vi "Set Tree Item Icon.vi"(0 "TreeControl in":refnum<vi>, 11 "error in (no error)":errorcluster) -> (4 "TreeControl out":refnum<vi>, 6 "Measurement folder Tags":string[](array[string]), 8 "Measurement file Tags":string[](array[string]), 15 "error out":errorcluster)   [LabVIEW 2021, in "Converter.lvlib"]
uses:
  Converter.lvlib
  0ae78c54-1542-49f1-a264-372c03cee13b.vi
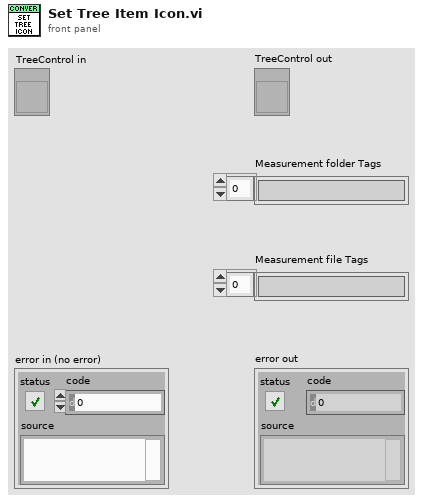
[diagram p1: front panel]
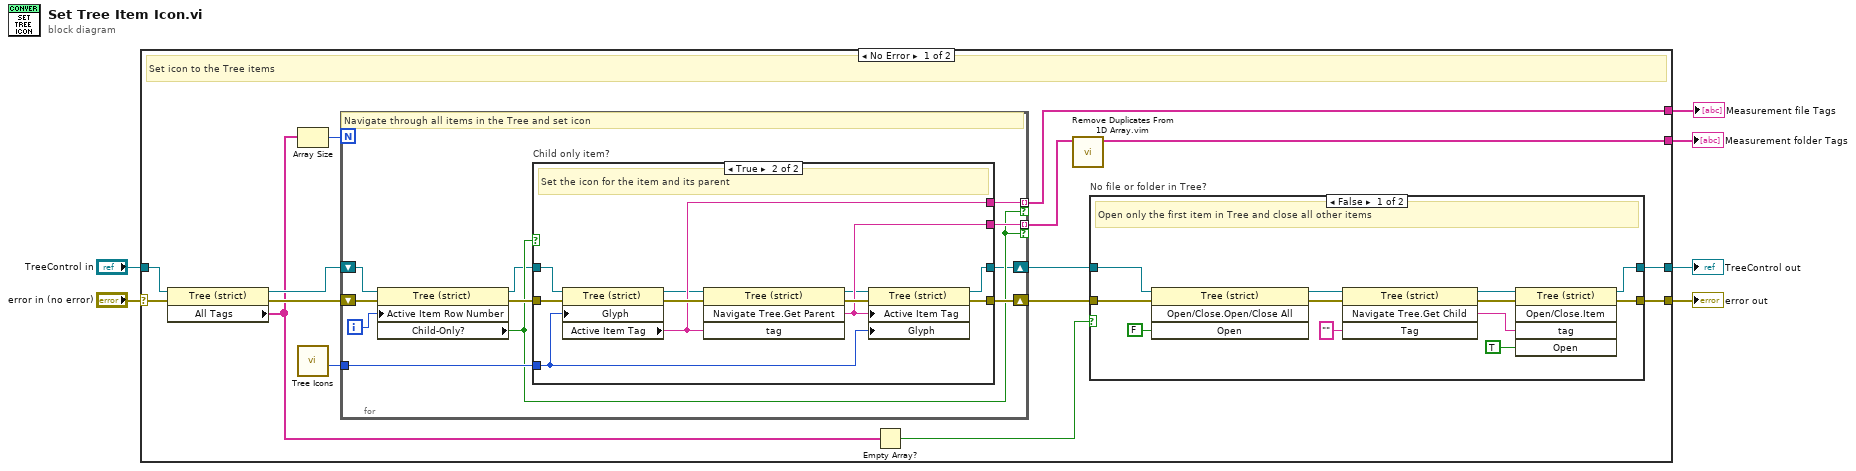
[diagram p0: block diagram]
diagram:
  n1 = case shown="No Error" "error in (no error)" {
    selector: "error in (no error)" -> [w20 w60]
    tunnel: "TreeControl in" -> [w21 w61]
    tunnel: [w11 w61] -> w4
    tunnel: [w12 w60] -> w3
    tunnel: [w16 _] -> w2
    tunnel: [w15 _] -> w1
    frame No Error {
      # "Set icon to the Tree items"
      n2 = property on="Property Node" class="Tree (strict)"(reference=w21, error in=w20) -> (reference out=w19:refnum<vi>, error out=w18:errorcluster, "All Tags"=w10:string[])
      n3 = Array Size(array=w10) -> (size(s)=w13:i32)
      n4 = call "Tree Icons.vi"() -> ("Not Selected"=w7:i32)  [unwired: 6 in, 1 out]
      n5 = for {
        N: w13 -> [_]
        shift-right: [w44] -> w14
        shift-left: w18 -> [w46]
        tunnel: w7 -> [w43]
        tunnel: [w42] -> w17 mode=indexing if=w40
        tunnel: [w41] -> w16 mode=indexing if=w40
        shift-right: [w36] -> w8
        shift-left: w19 -> [w37]
        i -> [w39]
        # "Navigate through all items in the Tree and set icon"
        n6 = property on="Property Node" class="Tree (strict)"(reference=w37, error in=w46, "Active Item Row Number"=w39) -> (reference out=w38:refnum<vi>, error out=w45:errorcluster, "Child-Only?"=w40:bool)
        n7 = case "Child only item?" shown="True" w40 {
          tunnel: w45 -> [w48 w59]
          tunnel: [w48 w56] -> w44
          tunnel: w43 -> [_ w55]
          tunnel: [_ w54] -> w42
          tunnel: [_ w53] -> w41
          tunnel: w38 -> [w47 w50]
          tunnel: [w47 w49] -> w36
          frame False {
            # "Pass"
          }
          frame True {
            # "Set the icon for the item and its parent"
            n8 = property on="Property Node" class="Tree (strict)"(reference=w50, error in=w59, "Glyph"=w55) -> (reference out=w52:refnum<vi>, error out=w58:errorcluster, "Active Item Tag"=w53:string)
            n9 = invoke on="Invoke Node" class="Tree (strict)" method="Navigate Tree.Get Parent"(reference=w52, error in=w58, "tag"=w53) -> (reference out=w51:refnum<vi>, error out=w57:errorcluster, "Navigate Tree:Get Parent"=w54:string)  [unwired: 1 in, 1 out]
            n10 = property on="Property Node" class="Tree (strict)"(reference=w51, error in=w57, "Active Item Tag"=w54, "Glyph"=w55) -> (reference out=w49:refnum<vi>, error out=w56:errorcluster)
          }
        }
      }
      n11 = Empty Array?(array=w10) -> (empty?=w9:bool)
      n12 = call "Remove Duplicates From 1D Array.vim"("array"=w17) -> ("array with duplicates removed"=w15:string[])  [unwired: 10 in]
      n13 = case "No file or folder in Tree?" shown="False" w9 {
        tunnel: w14 -> [w33 w35]
        tunnel: w8 -> [w31 w34]
        tunnel: [w26 w35] -> w12
        tunnel: [w22 w34] -> w11
        frame False {
          # "Open only the first item in Tree and close all other items"
          n14 = invoke class="Tree (strict)" method="Open/Close.Open/Close All"(reference=w31, error in=w33, "Open"=FALSE ("Open?")) -> (reference out=w28:refnum<vi>, error out=w32:errorcluster)  [unwired: 1 in, 2 out]
          n15 = invoke class="Tree (strict)" method="Navigate Tree.Get Child"(reference=w28, error in=w32, "Tag"="") -> (reference out=w25:refnum<vi>, error out=w29:errorcluster, "Navigate Tree:Get Child"=w24:string)  [unwired: 1 in, 1 out]
          n16 = invoke class="Tree (strict)" method="Open/Close.Item"(reference=w25, error in=w29, "tag"=w24, "Open"=TRUE ("Open?")) -> (reference out=w22:refnum<vi>, error out=w26:errorcluster)  [unwired: 1 in, 3 out]
        }
        frame True {
          # "Pass"
        }
      }
    }
    frame Error {
      # "Pass"
    }
  }
  "Measurement file Tags" <- w2
  "Measurement folder Tags" <- w1
  "TreeControl out" <- w4
  "error out" <- w3
